vi "Library - Methods.vi"(7 "Msg Chain":string, 8 "error in (no error)":errorcluster {"code" format="Error %.0f"}, 10 "Libraries":refnum<class "Library Documentation.lvclass">[](array[class]), 11 "VIDoc Printer - Confluence In":refnum<class "VIDoc Printer - Confluence.lvclass">) -> (0 "error out":errorcluster {"code" format="Error %.0f"}, 3 "VIDoc Printer - Confluence Out":refnum<class "VIDoc Printer - Confluence.lvclass">)   [LabVIEW 2023, in "VIDoc Printer - Confluence.lvlib" / "VIDoc Printer - Confluence.lvclass"]
uses:
  VIDoc Printer - Confluence.lvclass
  C:/projects/DMC/Tooling/Git-Action-Service/Source/Documentation Generation/Printers/Printer/VIDoc Printer.lvclass
  Parsing/Library Documentation/Library Documentation.lvclass
  Parsing/Library Documentation/Library Documentation.lvclass/Library Documentation.ctl
  Printer/VIDoc Printer.lvclass/VIDoc Printer.ctl
  Parsing/TypeDefs/VI Type Extended Enum.ctl
  Confluence Formatting/Types/Format Combo Box.ctl
  Types/VI Method Types.ctl
  VIDoc Printer - Confluence.lvclass/VIDoc Printer - Confluence.ctl
  Accessors/Get Library Methods Expand.vi
  Printer/Accessors/Get Library Settings - Methods Scope.vi
  Printer/Accessors/Get Library Settings - Methods Detail Level.vi
  Parsing/Library Documentation/Get LibMethods.vi
  Parsing/Library Documentation/Get Name.vi
  Printer/VIDoc Printer.lvclass
  UI Interaction/UI Interaction.lvclass
  Parsing/VIDoc Parsing.lvlib
  Confluence Formatting/Confluence Formatting.lvlib
  C:/projects/DMC/Tooling/Git-Action-Service/Source/Documentation Generation/Printers/Confluence Printer/VIDoc Printer - Confluence.lvclass
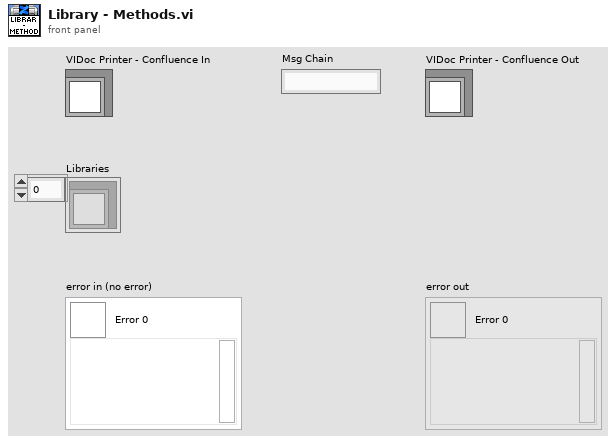
[diagram p1: front panel]
types:
  T1 = typedef "VIDoc Parsing.lvlib/VI Type Extended Enum.ctl" = enum16{"Unknown", "Class Method", "Class Accessor Get", "Class Accessor Set", "Class Control", "Library Method", "Library Control", "VI", "Control"}
  T2 = typedef "VIDoc Printer - Confluence.lvlib/VIDoc Printer - Confluence.lvclass/VI Method Types.ctl" = enum16{"Library", "Class", "Interface", "LLB", "UI", "List"}
  T3 = typedef "Confluence Formatting.lvlib/Format Combo Box.ctl" = string
  T4 = typedef "VIDoc Parsing.lvlib/Method Spec Cluster.ctl" = cluster{"VI Type Ext":T1, "Name":string, "Path":path, "Get Conpane Image":T5, "Description":string, "Get Library Access Scope":enum32{"invalid scope", "public", "private", "protected", "community"}, "Dispatch":T6, "ContainsCompiledCode":bool, "Exec.IsReentrant":bool, "Exec.ReentrancyType":enum16{"Share clones between instances", "Preallocate clone for each instance"}, "ExecInlining":bool, "ExecInlineIfPossible":bool, "Auto Err Handling":bool, "CodeComplexity":sgl, "Bookmark Tags":string[], "Control VI Type":enum32{"not a control VI", "control", "typedef", "strict typedef"}, "Controls":T7[], "VI Type":enum32{"invalid VI type", "Standard VI", "Control VI", "Global VI", "Polymorphic VI", "Configuration VI", "SubSystem", "Facade VI", "Method VI", "Statechart Diagram VI"}, "Minimum Size":T9, "Front Panel Window:Title":string, "Front Panel Window:Behavior":enum32{"Invalid", "Default", "Floating", "Floating/Auto-Hide", "Modal"}, "Front Panel Window:Closeable":bool, "Must Override":bool, "Must Use Parent Implementation":bool, "VI Icon":T5, "Front Panel":T5, "History:Revision Number":u32, "Metrics:Total Data Size":u32, "Execution:Allow Debugging":bool, "Execution:Preferred Exec System":enum32{"invalid execution system", "user interface", "standard", "instrument i/o", "data acquisition", "other 1", "other 2", "same as caller"}, "Execution:Priority":enum32{"invalid priority", "background priority", "normal priority", "above normal priority", "high priority", "time critical priority", "subroutine"}, "BM Tag Text":string[], "Block Diagram":T5, "Structure Tree":T10[]}
  T5 = typedef "imagedata.ctl" = cluster{"image type":i32, "image depth":i32, "image":u8[], "mask":u8[], "colors":u32[], "Rectangle":cluster{"left":i16, "top":i16, "right":i16, "bottom":i16}}
  T6 = typedef "VIDoc Parsing.lvlib/Class Dispatch Type Enum.ctl" = enum16{"None", "Static", "Dynamic"}
  T7 = typedef "VIDoc Parsing.lvlib/Controls Info Cluster.ctl" = cluster{"Name":string, "Description":string, "Data Type":string, "Tip Strip":string, "UID":i32, "Image Data":T5, "ToggleKeyBind":T8, "Raw Label":string, "Raw Caption":string}
  T8 = typedef "LVKeyTypeDef.ctl" = cluster{"Focus":bool, "Control":bool, "Shift":bool, "Key":string}
  T9 = typedef "LVPointTypeDef.ctl" = cluster{"Horizontal":i16, "Vertical":i16}
  T10 = typedef "VIDoc Parsing.lvlib/Structure Reporter.lvlib/Tree Cluster.ctl" = cluster{"Object Class Name":string, "Labels":string[], "Child Tag":string, "Item Indent":i32, "Child Only?":bool, "Glyph Index":i32}
  T11 = typedef "VIDoc Printer.lvlib/Printer Settings.lvclass/Scope Settings.ctl" = cluster{"Public":bool, "Protected":bool, "Community":bool, "Private":bool, "Unknown":bool}
  T12 = typedef "VIDoc Printer.lvlib/Printer Settings.lvclass/Detail Level Enum.ctl" = enum16{"None", "Minimal", "Standard", "Full"}
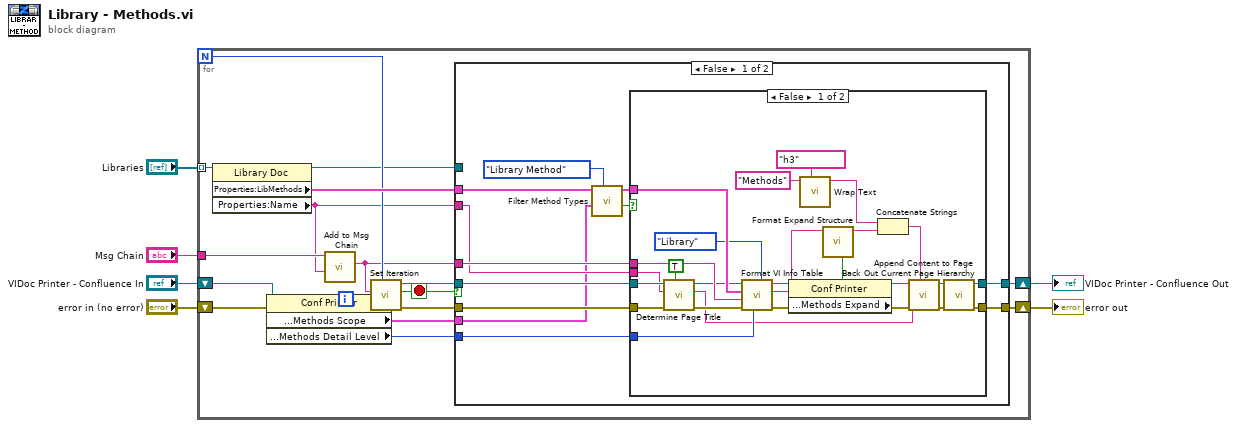
[diagram p0: block diagram]
diagram:
  n1 = for {
    N -> [w18]
    shift-right: [w23] -> w6
    shift-left: "error in (no error)" -> [w21]
    shift-right: [w24] -> w5
    shift-left: "VIDoc Printer - Confluence In" -> [w11]
    tunnel: "Libraries" -> [w25] mode=indexing
    tunnel: "Msg Chain" -> [w16]
    i -> [w17]
    stop <- w14 stop-if-true
    n2 = property class="Library Doc"(reference=w25) -> (reference out=w13:refnum<class "Library Documentation.lvclass">, "Properties:LibMethods"=w22:T4[], "Properties:Name"=w15:string)  [unwired: 1 in, 1 out]
    n3 = property class="Conf Printer"(reference=w11, error in=w21) -> (reference out=w10:refnum<class "VIDoc Printer - Confluence.lvclass">, error out=w12:errorcluster, "Properties:Settings:Libraries:Methods Scope"=w8:T11, "Properties:Settings:Libraries:Methods Detail Level"=w7:T12)
    n4 = call "Add to Msg Chain.vi"("New"=w15, "Msg Chain in"=w16) -> ("Msg Chain out"=w9:string)  [unwired: 9 in]
    n5 = call "Set Iteration.vi"("Progress Max"=w18, "error in (no error)"=w12, "Progress Value"=w17, "Message (No Message Update)"=w9, "VIDoc Printer In"=w10) -> ("error out"=w19:errorcluster, "Abort?"=w14:bool, "VIDoc Printer Out"=w20:refnum<class "VIDoc Printer - Confluence.lvclass">)  [unwired: 4 in]
    n6 = case shown="False" w14 {
      tunnel: [w37 w65] -> w24
      tunnel: [w36 w66] -> w23
      tunnel: w22 -> [w31 _]
      tunnel: w20 -> [w34 w65]
      tunnel: w19 -> [w35 w66]
      tunnel: w15 -> [w32 _]
      tunnel: w13 -> [_ _]
      tunnel: w9 -> [w33 _]
      tunnel: w8 -> [w27 _]
      tunnel: w7 -> [w26 _]
      frame False {
        n7 = call "Filter Method Types.vi"("VI Type to filter for"=VI_Type_Extended_Enum."Library Method" ("y"), "Scope"=w27, "Methods"=w31) -> ("All Filtered?"=w29:bool, "Filtered Methods"=w30:T4[])  [unwired: 6 in, 1 out]
        n8 = case shown="False" w29 {
          tunnel: [w44 w64] -> w37
          tunnel: [w46 w63] -> w36
          tunnel: w35 -> [w49 w63]
          tunnel: w34 -> [w51 w64]
          tunnel: w33 -> [w55 _]
          tunnel: w26 -> [w54 _]
          tunnel: w30 -> [w52 _]
          tunnel: w32 -> [w42 _]
          frame False {
            n9 = call "Determine Page Title.vi"("Update Current Page (F)"=TRUE, "error in (no error)"=w49, "Name"=w42, "VIDoc Printer - Confluence In"=w51) -> ("error out"=w48:errorcluster, "Page Title"=w43:string, "VIDoc Printer - Confluence Out"=w50:refnum<class "VIDoc Printer - Confluence.lvclass">)  [unwired: 4 in, 1 out]
            n10 = call "Format VI Info Table.vi"("Type"=VI_Method_Types."Library", "Methods"=w54, "Error in"=w48, "Msg Chain"=w55, "VI Info Array"=w52, "VIDoc Printer - Confluence In"=w50) -> ("Error out"=w57:errorcluster, "Table String"=w53:string, "VIDoc Printer - Confluence Out"=w56:refnum<class "VIDoc Printer - Confluence.lvclass">)  [unwired: 3 in]
            n11 = property class="Conf Printer"(reference=w56) -> (reference out=w40:refnum<class "VIDoc Printer - Confluence.lvclass">, "Properties:Expand?:Library:Methods Expand"=w39:bool)  [unwired: 1 in, 1 out]
            n12 = call "Wrap Text.vi"("Formatting"=T3 "h3", "String"="Methods") -> ("Wrapped String"=w59:string)  [unwired: 8 in, 1 out]
            n13 = call "Format Expand Structure.vi"("Enable? (T)"=w39, "Content"=w53) -> ("Expand String"=w41:string)  [unwired: 8 in, 1 out]
            n14 = Concatenate Strings(w59, w41) -> (w58:string)
            n15 = call "Append Content to Page.vi"("Page Content"=w58, "error in (no error)"=w57, "Page Title"=w43, "VIDoc Printer - Confluence In"=w40) -> ("error out"=w62:errorcluster, "VIDoc Printer - Confluence Out"=w45:refnum<class "VIDoc Printer - Confluence.lvclass">)  [unwired: 6 in]
            n16 = call "Back Out Current Page Hierarchy.vi"("error in (no error)"=w62, "VIDoc Printer - Confluence In"=w45) -> ("error out"=w46:errorcluster, "VIDoc Printer - Confluence Out"=w44:refnum<class "VIDoc Printer - Confluence.lvclass">)  [unwired: 8 in]
          }
          frame True {
          }
        }
      }
      frame True {
      }
    }
  }
  "error out" <- w6
  "VIDoc Printer - Confluence Out" <- w5
